vi "Pre Launch Init.vi"(11 "cRIO-CO2 in":refnum<class "cRIO-CO2.lvclass">) -> (0 "error out":errorcluster, 3 "cRIO-CO2 out":refnum<class "cRIO-CO2.lvclass">)   [LabVIEW 2015, in "cRIO-Carbondioxide.lvlib" / "cRIO-CO2.lvlib" / "cRIO-CO2.lvclass"]
doc: "(<B>Filename</B>: Actor Framework.lvlib:Actor.lvclass:Pre Launch Init.vi)\n\nDefines behavior that occurs after the Launch Actor method is invoked but before the actor's Actor Core method begins running.\n\nThe Pre Launch Init method is guaranteed to finish before the Launch Actor method returns to its caller and before the actor itself receives any messages. Any references that the Pre Launch Init method obtains are guaranteed to have the same lifetime as the actor itself. Any errors that the Pre Launch Init method returns will abort the launch.\n\nBy default, this method does nothing. A descendant class may override it to define behavior."
uses:
  cRIO-CO2.lvclass
  <vilib>/ActorFramework/Actor/Actor.lvclass/Actor.ctl
  <vilib>/ActorFramework/Message Enqueuer/Message Enqueuer.lvclass/Message Enqueuer.ctl
  Controls/Dedicated Enqueuers.ctl
  <vilib>/ActorFramework/Message Enqueuer/Message Enqueuer.lvclass
  Controls/Sample Transfer Assignment.ctl
  Controls/Sample Transfer Container Enumerator.ctl
  cRIO-CO2 Messages/Timeout Msg/Timeout Msg.lvclass
  Controls/Vacuum State Cluster.ctl
  Controls/Vacuum State Enumerator.ctl
  cRIO-CO2.lvclass/cRIO-CO2.ctl
  cRIO-CO2 Messages/Log Message Msg/Log Message Msg.lvclass/Log Message Msg.ctl
  cRIO-CO2 Messages/Launch He Line Msg/Launch He Line Msg.lvclass/Launch He Line Msg.ctl
  cRIO-CO2 Messages/Sample Push Reset to Idle Msg/Sample Push Reset to Idle Msg.lvclass/Sample Push Reset to Idle Msg.ctl
  cRIO-CO2 Messages/Sample Transfer Reset to Idle Msg/Sample Transfer Reset to Idle Msg.lvclass/Sample Transfer Reset to Idle Msg.ctl
  <vilib>/ActorFramework/Message Enqueuer/Init from Existing Queue.vi
  <vilib>/ActorFramework/Message Enqueuer/Enqueue.vi
  <vilib>/ActorFramework/Message Priority Queue/Priority Enqueue.vi
  cRIO-CO2 Messages/Sample Transfer Reset to Idle Msg/Sample Transfer Reset to Idle Msg.lvclass
  cRIO-CO2 Messages/Sample Push Reset to Idle Msg/Sample Push Reset to Idle Msg.lvclass
  cRIO-CO2 Messages/Launch Cylinder Msg/Launch Cylinder Msg.lvclass
  cRIO-CO2 Messages/Launch Transfer Line Msg/Launch Transfer Line Msg.lvclass
  cRIO-CO2 Messages/Launch He Line Msg/Launch He Line Msg.lvclass
  Interlocks/Interlock Chain/Interlock Chain.lvclass
  cRIO-CO2 Messages/Launch Turbo Msg/Launch Turbo Msg.lvclass
  cRIO-CO2 Messages/Launch Preparation Line Msg/Launch Preparation Line Msg.lvclass
  cRIO-CO2 Messages/Launch Syringe Line Msg/Launch Syringe Line Msg.lvclass
  cRIO-CO2 Messages/Launch Capillary Line Msg/Launch Capillary Line Msg.lvclass
  cRIO-CO2 Messages/Launch Storage Line Msg/Launch Storage Line Msg.lvclass
  cRIO-CO2 Messages/Launch Sample Line Msg/Launch Sample Line Msg.lvclass
  cRIO-CO2 Messages/Launch Vacuum Msg/Launch Vacuum Msg.lvclass
  cRIO-CO2 Messages/Log Message Msg/Log Message Msg.lvclass
  <vilib>/ActorFramework/Actor/Actor.lvclass
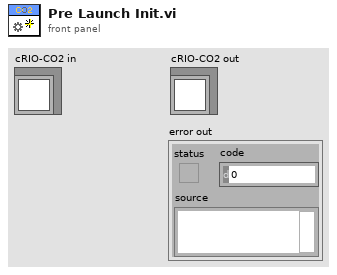
[diagram p1: front panel]
types:
  T1 = typedef "Vacuum State Cluster.ctl" = cluster{"Vacuum State":T2, "Pressure":dbl, "Raw Pressure":dbl, "d/dt":dbl}
  T2 = typedef "Vacuum State Enumerator.ctl" = enum16{"Pressure Rising", "Plateau", "Pressure Dropping", "Valley", "Low Valley", "Leak", "Unknown"}
  T3 = typedef "Sample Transfer Assignment.ctl" = cluster{"Source":T4, "Target":T4}
  T4 = typedef "Sample Transfer Container Enumerator.ctl" = enum16{"None", "Sample 1", "Sample 2", "Sample 3", "Sample 4", "Sample 5", "Storage 01", "Storage 02", "Storage 03", "Storage 04", "Storage 05", "Storage 06", "Storage 07", "Storage 08", "Storage 09", "Storage 10", "Storage 11", "Storage 12", "Syringe", "Undefined"}
  T5 = typedef "Dedicated Enqueuers.ctl" = cluster{"Freezers":cluster{"Syringe":refnum<class "Message Enqueuer.lvclass">, "Tank 1":refnum<class "Message Enqueuer.lvclass">, "Tank 2":refnum<class "Message Enqueuer.lvclass">, "Tank 3":refnum<class "Message Enqueuer.lvclass">, "Tank 4":refnum<class "Message Enqueuer.lvclass">}, "Heaters":cluster{"Syringe":refnum<class "Message Enqueuer.lvclass">, "Piston":refnum<class "Message Enqueuer.lvclass">}, "Blowers":cluster{"Tank 1":refnum<class "Message Enqueuer.lvclass">, "Tank 2":refnum<class "Message Enqueuer.lvclass">, "Tank 3":refnum<class "Message Enqueuer.lvclass">, "Tank 4":refnum<class "Message Enqueuer.lvclass">, "Syringe":refnum<class "Message Enqueuer.lvclass">}, "Sample Line":refnum<class "Message Enqueuer.lvclass">, "Storage Line":refnum<class "Message Enqueuer.lvclass">, "Transfer Line":refnum<class "Message Enqueuer.lvclass">, "Syringe Stepper":refnum<class "Message Enqueuer.lvclass">, "Syringe Line":refnum<class "Message Enqueuer.lvclass">, "Capillary Line":refnum<class "Message Enqueuer.lvclass">, "Preparation Line":refnum<class "Message Enqueuer.lvclass">, "Turbo":refnum<class "Message Enqueuer.lvclass">, "Vacuum":refnum<class "Message Enqueuer.lvclass">, "He Line":refnum<class "Message Enqueuer.lvclass">, "Cylinder":refnum<class "Message Enqueuer.lvclass">}
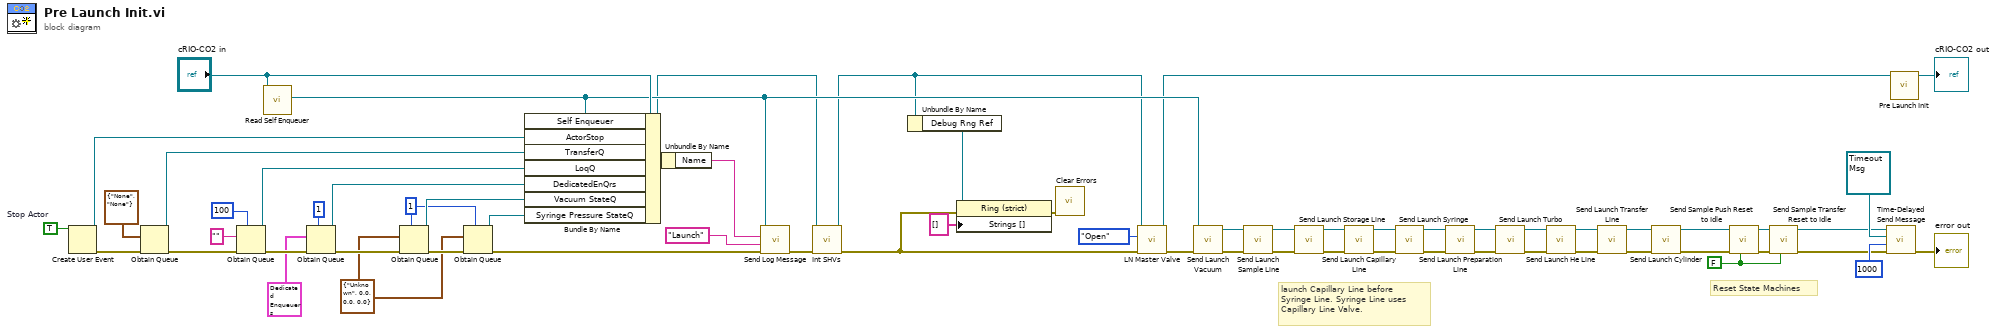
[diagram p0: block diagram]
diagram:
  w6 = FALSE ("Echo (True)")
  w18 = T1 {"Vacuum State"=enum."Unknown", "Pressure"=0.0, "Raw Pressure"=0.0, "d/dt"=0.0} ("Vacuum State Cluster")
  w15 = 1 ("max queue size (-1, unlimited)")
  w55 = TRUE  # Stop Actor
  # "Reset State Machines"
  # "launch Capillary Line before\nSyringe Line. Syringe Line uses\nCapillary Line Valve."
  n1 = Create User Event(user event datatype=w55) -> (user event=w54:refnum<user-event>, error out=w39:errorcluster)  [unwired: 1 in]
  n2 = Obtain Queue(element data type=T3 {"Source"=enum."None", "Target"=enum."None"} ("Transfer Assignment"), error in (no error)=w39) -> (queue out=w37:refnum<queue>, error out=w38:errorcluster)  [unwired: 3 in, 1 out]
  n3 = Obtain Queue(max queue size (-1, unlimited)=100, element data type="", error in (no error)=w38) -> (queue out=w45:refnum<queue>, error out=w44:errorcluster)  [unwired: 2 in, 1 out]
  n4 = call <vilib>:"Read Self Enqueuer.vi"("Actor"="cRIO-CO2 in") -> ("Self Enqueuer"=w31:refnum<class "Message Enqueuer.lvclass">)  [unwired: 10 in]
  n5 = Obtain Queue(max queue size (-1, unlimited)=1, element data type=T5 {"Freezers"={"Syringe"=refnum, "Tank 1"=refnum, "Tank 2"=refnum, "Tank 3"=refnum, "Tank 4"=refnum}, "Heaters"={"Syringe"=refnum, "Piston"=refnum}, "Blowers"={"Tank 1"=refnum, "Tank 2"=refnum, "Tank 3"=refnum, "Tank 4"=refnum, "Syringe"=refnum}, "Sample Line"=refnum, "Storage Line"=refnum, "Transfer Line"=refnum, "Syringe Stepper"=refnum, "Syringe Line"=refnum, "Capillary Line"=refnum, "Preparation Line"=refnum, "Turbo"=refnum, "Vacuum"=refnum, "He Line"=refnum, "Cylinder"=refnum} ("Dedicated Enqueuers"), error in (no error)=w44) -> (queue out=w33:refnum<queue>, error out=w25:errorcluster)  [unwired: 2 in, 1 out]
  n6 = Obtain Queue(max queue size (-1, unlimited)=w15, element data type=w18, error in (no error)=w25) -> (queue out=w24:refnum<queue>, error out=w19:errorcluster)  [unwired: 2 in, 1 out]
  n7 = Obtain Queue(max queue size (-1, unlimited)=w15, element data type=w18, error in (no error)=w19) -> (queue out=w17:refnum<queue>, error out=w16:errorcluster)  [unwired: 2 in, 1 out]
  n8 = Bundle By Name(cluster="cRIO-CO2 in", "Self Enqueuer"=w31, "ActorStop"=w54, "TransferQ"=w37, "LoqQ"=w45, "DedicatedEnQrs"=w33, "Vacuum StateQ"=w24, "Syringe Pressure StateQ"=w17) -> (w26:refnum<class "cRIO-CO2.lvclass">)
  n9 = Unbundle By Name(w26) -> ("Name"=w58:string)
  n10 = call "Send Log Message.vi"("error in (no error)"=w16, "String"="Launch", "Source Name"=w58, "Message Enqueuer"=w31) -> ("error out"=w53:errorcluster)  [unwired: 6 in, 1 out]
  n11 = call "Int SHVs.vi"("error in (no error)"=w53, "cRIO-CO2 in"=w26) -> ("error out"=w5:errorcluster, "cRIO-CO2 out"=w3:refnum<class "cRIO-CO2.lvclass">)  [unwired: 8 in]
  n12 = Unbundle By Name(w3) -> ("Debug Rng Ref"=w57:refnum<vi>)
  n13 = property class="Ring (strict)"(reference=w57, error in=w5, "Strings []"=string[] []) -> (error out=w52:errorcluster)  [unwired: 1 out]
  n14 = call <vilib>:"Clear Errors.vi"("error in (no error)"=w52) -> ()  [unwired: 5 in, 2 out]
  n15 = call "LN Master Valve.vi"("error in (no error)"=w5, "Action (Read State)"=enum16{"Read State", "Open", "Close"}."Open", "cRIO-CO2 in"=w3) -> ("error out"=w4:errorcluster, "cRIO-CO2 out"=w2:refnum<class "cRIO-CO2.lvclass">)  [unwired: 6 in, 1 out]
  n16 = call "Send Launch Vacuum.vi"("error in (no error)"=w4, "Message Enqueuer"=w31) -> ("error out"=w32:errorcluster, "Message Enqueuer out"=w30:refnum<class "Message Enqueuer.lvclass">)  [unwired: 8 in]
  n17 = call "Send Launch Sample Line.vi"("error in (no error)"=w32, "Message Enqueuer"=w30) -> ("error out"=w51:errorcluster, "Message Enqueuer out"=w50:refnum<class "Message Enqueuer.lvclass">)  [unwired: 8 in]
  n18 = call "Send Launch Storage Line.vi"("error in (no error)"=w51, "Message Enqueuer"=w50) -> ("error out"=w34:errorcluster, "Message Enqueuer out"=w35:refnum<class "Message Enqueuer.lvclass">)  [unwired: 8 in]
  n19 = call "Send Launch Capillary Line.vi"("error in (no error)"=w34, "Message Enqueuer"=w35) -> ("error out"=w48:errorcluster, "Message Enqueuer out"=w49:refnum<class "Message Enqueuer.lvclass">)  [unwired: 8 in]
  n20 = call "Send Launch Syringe.vi"("error in (no error)"=w48, "Message Enqueuer"=w49) -> ("error out"=w47:errorcluster, "Message Enqueuer out"=w46:refnum<class "Message Enqueuer.lvclass">)  [unwired: 8 in]
  n21 = call "Send Launch Preparation Line.vi"("error in (no error)"=w47, "Message Enqueuer"=w46) -> ("error out"=w41:errorcluster, "Message Enqueuer out"=w40:refnum<class "Message Enqueuer.lvclass">)  [unwired: 8 in]
  n22 = call "Send Launch Turbo.vi"("error in (no error)"=w41, "Message Enqueuer"=w40) -> ("error out"=w22:errorcluster, "Message Enqueuer out"=w23:refnum<class "Message Enqueuer.lvclass">)  [unwired: 8 in]
  n23 = call "Send Launch He Line.vi"("error in (no error)"=w22, "Message Enqueuer"=w23) -> ("error out"=w21:errorcluster, "Message Enqueuer out"=w20:refnum<class "Message Enqueuer.lvclass">)  [unwired: 8 in]
  n24 = call "Send Launch Transfer Line.vi"("error in (no error)"=w21, "Message Enqueuer"=w20) -> ("error out"=w13:errorcluster, "Message Enqueuer out"=w14:refnum<class "Message Enqueuer.lvclass">)  [unwired: 8 in]
  n25 = call "Send Launch Cylinder.vi"("error in (no error)"=w13, "Message Enqueuer"=w14) -> ("error out"=w10:errorcluster, "Message Enqueuer out"=w12:refnum<class "Message Enqueuer.lvclass">)  [unwired: 8 in]
  n26 = call "Send Sample Push Reset to Idle.vi"("Echo (True)"=w6, "error in (no error)"=w10, "Message Enqueuer"=w12) -> ("error out"=w9:errorcluster, "Message Enqueuer out"=w11:refnum<class "Message Enqueuer.lvclass">)  [unwired: 7 in]
  n27 = call "Send Sample Transfer Reset to Idle.vi"("Echo (True)"=w6, "error in (no error)"=w9, "Message Enqueuer"=w11) -> ("error out"=w8:errorcluster, "Message Enqueuer out"=w7:refnum<class "Message Enqueuer.lvclass">)  [unwired: 7 in]
  n28 = call <vilib>:"Time-Delayed Send Message.vi"("error in (no error)"=w8, "Milliseconds To Wait"=1000, "Message"=refnum<class "Timeout Msg.lvclass"> refnum ("cRIO-Carbondioxide.lvlib:cRIO-CO2.lvlib:Timeout Msg.lvclass"), "Message Enqueuer"=w7) -> ("error out"=→"error out":errorcluster)  [unwired: 6 in, 1 out]
  n29 = call-parent "Pre Launch Init.vi"("Actor in"=w2) -> ("Actor out"=→"cRIO-CO2 out":refnum<class "cRIO-CO2.lvclass">)  [unwired: 9 in, 1 out]
